vi "Configure Comparator SLIM.vi"(8 "error in (no error)":errorcluster, 9 "High Limit Value (0)":dbl, 10 "Low Limit Value (0)":dbl, 11 "VISA resource name":refnum<visa-resource-name>) -> (0 "error out":errorcluster, 3 "VISA resource name out":refnum<visa-resource-name>)   [LabVIEW 2014, in "LCR Meter.lvlib"]
doc: "Sets the LOW/HIGH limit value for the secondary parameter."
uses:
  <instrlib>/LCR Meter/Examples/LCR Meter Acquire Single_1 Folder/LCR Meter.lvlib
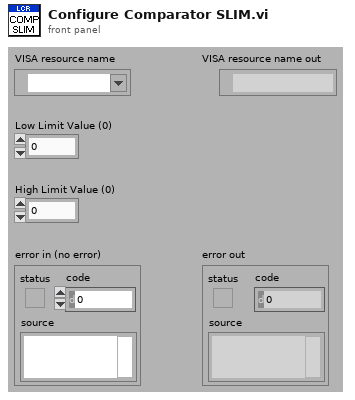
[diagram p1: front panel]
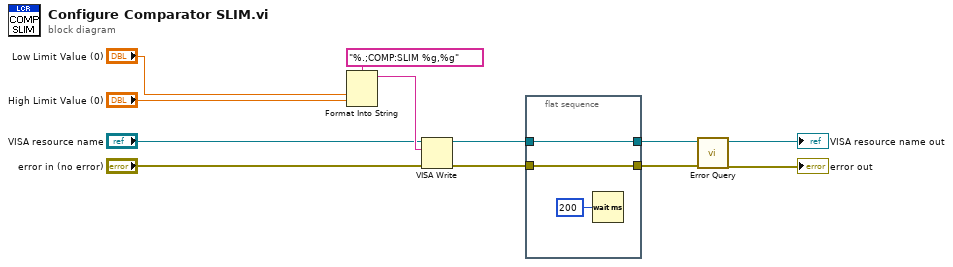
[diagram p0: block diagram]
diagram:
  n1 = Format Into String(format string="%.;COMP:SLIM %g,%g", "Low Limit Value (0)", "High Limit Value (0)") -> (resulting string=w9:string)  [unwired: 2 in, 1 out]
  n2 = VISA Write(VISA resource name="VISA resource name", write buffer=w9, error in (no error)="error in (no error)") -> (VISA resource name out=w4:refnum<visa-resource-name>, error out=w2:errorcluster)  [unwired: 1 out]
  n3 = flat-sequence {
    tunnel: w4 -> [w15]
    tunnel: [w15] -> w3
    tunnel: w2 -> [w14]
    tunnel: [w14] -> w1
    frame #0 {
      n4 = Wait (ms)(milliseconds to wait=u32 200) -> ()  [unwired: 1 out]
    }
  }
  n5 = call <instrlib>:"Error Query.vi"("error in (no error)"=w1, "VISA resource name"=w3) -> ("error out"=→"error out":errorcluster, "VISA resource name out"=→"VISA resource name out":refnum<visa-resource-name>)  [unwired: 6 in, 2 out]
